vi "Get SLSC Module GUID.vi"(8 "error in (no error)":errorcluster, 11 "SLSC Module":u64) -> (0 "error out":errorcluster, 2 "Module GUID":string, 3 "SLSC Module out":u64)   [LabVIEW 2019, in "VeriStand SLSC Scripting.lvlib"]
uses:
  VeriStand SLSC Scripting.lvlib
  NationalInstruments.VeriStand.SystemDefinitionAPI
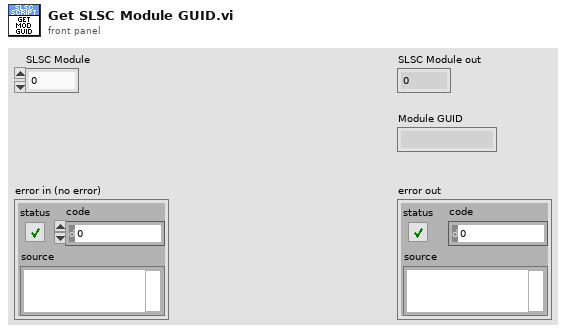
[diagram p1: front panel]
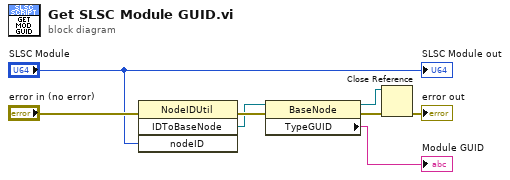
[diagram p0: block diagram]
diagram:
  n1 = invoke class="NodeIDUtil" method="IDToBaseNode"(error in="error in (no error)", "nodeID"="SLSC Module") -> (error out=w7:errorcluster, "IDToBaseNode"=w4:refnum<k24>)  [unwired: 2 in, 2 out]
  n2 = property class="BaseNode"(reference=w4, error in=w7) -> (reference out=w5:refnum<k24>, error out=w6:errorcluster, "TypeGUID"=→"Module GUID":string)
  n3 = Close Reference(reference=w5, error in (no error)=w6) -> (error out=→"error out":errorcluster)
  "SLSC Module out" <- "SLSC Module"
